vi "FPGA_RW_Vars.vi"() -> ()   [LabVIEW 2019]
panel:
  out "Temperature 2 (NI-9219)":T1
  out "Temperature (NI-9219)":T1
  in  "Stop":bool
  out "Error Out":errorcluster
  out "Reading?":bool
  out "Vibration (NI-9234)":T2
  out "Voltage (NI-9225)":cluster{"Voltage (CH0)":waveform(dbl)}
  out "Voltage (NI-9215)":T3
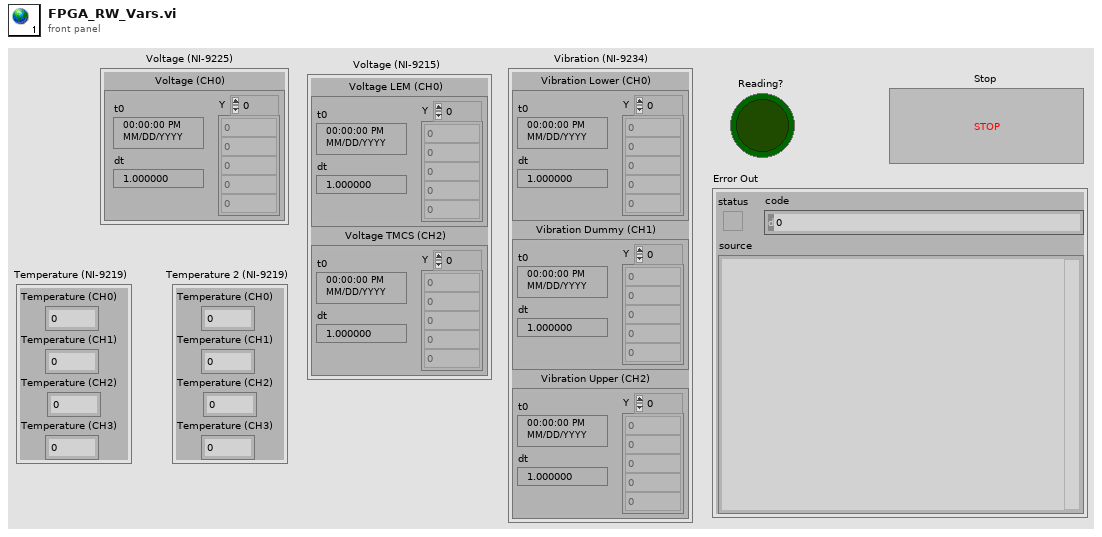
[diagram p1: front panel]
types:
  T1 = cluster{"Temperature (CH0)":dbl, "Temperature (CH1)":dbl, "Temperature (CH2)":dbl, "Temperature (CH3)":dbl}
  T2 = cluster{"Vibration Lower (CH0)":waveform(dbl), "Vibration Dummy (CH1)":waveform(dbl), "Vibration Upper (CH2)":waveform(dbl)}
  T3 = cluster{"Voltage LEM (CH0)":waveform(dbl), "Voltage TMCS (CH2)":waveform(dbl)}
diagram:
